vi "Message to Other Guardian.vi"(0 "Guardian in":refnum<class "Guardian.lvclass">, 5 "Guardian ID":string, 7 "Message":string, 9 "Data":variant, 11 "error in (no error)":errorcluster) -> (4 "Guardian out":refnum<class "Guardian.lvclass">, 15 "error out":errorcluster)   [LabVIEW 2026, in "TALOS.lvlib" / "Guardian.lvlib" / "Guardian.lvclass"]
uses:
  Guardian.lvclass
  C:/LabVIEW Code/TALOS/talos/Ancestor/Ancestor/Ancestor.lvclass
  Ancestor/Ancestor/Ancestor.lvclass/Ancestor.ctl
  Ancestor/Ancestor/Read ID.vi
  Support VIs/Generate Error.vi
  FGV/Error Memory/Get Error Description.vi
  Support VIs/Get PC name.vi
  Support VIs/Get Class Name.vi
  <vilib>/Utility/error.llb/Clear Errors.vi
  FGV/Error Memory/Error Memory Core.vi
  <vilib>/AdvancedString/Delimited String to 1D String Array.vi
  <vilib>/AdvancedString/Delimited String to 1D String Array (string).vi
  Support VIs/Circus Root Path.vi
  FGV/Error Memory/Error Crt Lvl checker.vi
  FGV/Error Memory/Error Memory Core.vi/40c8088d-b597-4017-91af-faa98e00292e.vi
  FGV/Error Memory/Error Memory Core.vi/d4a3ab98-063c-4e44-b43d-fbdcfe6c2be2.vi
  Support VIs/Global Memory.vi
  <vilib>/Utility/LVClass/Get LV Class Name.vi
  Support VIs/Is in Packed Library.vi
  Support VIs/TALOS Root path.vi
  Support VIs/Read CSV worksheet.vi
  Support VIs/Global Constants.vi
  <vilib>/Utility/error.llb/General Error Handler.vi
  Support VIs/Error Log.vi
  Ancestor/Ancestor/Ancestor.lvclass
  <vilib>/Comparison/Equal/Equal Functor/Equal Functor.lvclass
  TALOS.lvlib
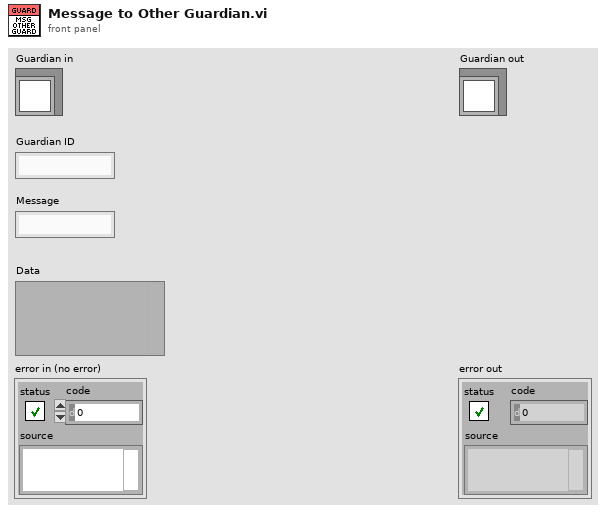
[diagram p1: front panel]
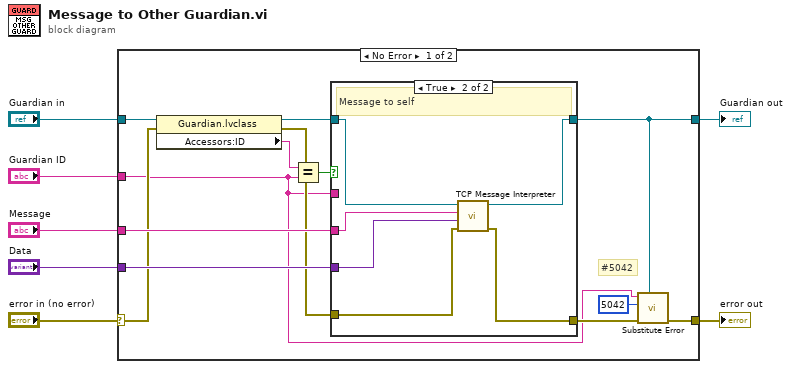
[diagram p0: block diagram]
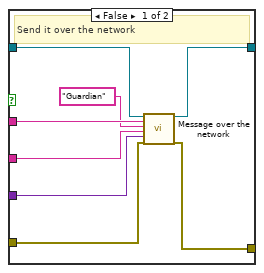
[diagram p2: hidden frame]
diagram:
  n1 = case shown="No Error" "error in (no error)" {
    selector: "error in (no error)" -> [w18 w36]
    tunnel: [w11 w36] -> w6
    tunnel: [w10 w35] -> w4
    tunnel: "Guardian in" -> [w17 w35]
    tunnel: "Guardian ID" -> [w8 _]
    tunnel: "Message" -> [w20 _]
    tunnel: "Data" -> [w19 _]
    frame No Error {
      # "#5042"
      n2 = property class="Guardian.lvclass"(reference=w17, error in=w18) -> (reference out=w14:refnum<class "Guardian.lvclass">, error out=w13:errorcluster, "Accessors:ID"=w16:string)
      n3 = Equal?(x=w16, y=w8) -> (x = y?=w15:bool)
      n4 = case shown="True" w15 {
        tunnel: w14 -> [w27 w34]
        tunnel: w13 -> [w22 w30]
        tunnel: w20 -> [w24 w33]
        tunnel: w19 -> [w23 w32]
        tunnel: [w28 w31] -> w10
        tunnel: [w21 w29] -> w12
        tunnel: w8 -> [w26 _]
        frame False {
          # "Send it over the network"
          n5 = call "Message over the network.vi"("Guardian in"=w27, "Destination GD ID"=w26, "Target ID (uService ID or \"Guardian\")"="Guardian" ("Target ID (uService ID or \"Guardian\")"), "Message"=w24, "Data"=w23, "error in (no error)"=w22) -> ("Guardian out"=w28:refnum<class "Guardian.lvclass">, "error out"=w21:errorcluster)  [unwired: 12 in]
        }
        frame True {
          # "Message to self"
          n6 = call "TCP Message Interpreter.vi"("error in (no error)"=w30, "Data"=w32, "Message"=w33, "Guardian in"=w34) -> ("error out"=w29:errorcluster, "Guardian out"=w31:refnum<class "Guardian.lvclass">)  [unwired: 6 in]
        }
      }
      n7 = call "Substitute Error.vi"("LabVIEW Object"=w10, "error in (no error)"=w12, "Error Code"=5042, "Optional String"=w8) -> ("error out"=w11:errorcluster)  [unwired: 7 in]
    }
    frame Error {
    }
  }
  "error out" <- w6
  "Guardian out" <- w4
